vi "ClassPanel.vi"(8 "error in (no error)":errorcluster caption="entrée d'erreur (pas d'erreur)", 11 "SymphonyCCD.lvclass":refnum<class "SymphonyCCD.lvclass">) -> (0 "error out":errorcluster caption="sortie d'erreur", 3 "SymphonyCCD.lvclass Out":refnum<class "SymphonyCCD.lvclass">)   [LabVIEW 2019, in "SymphonyCCD.lvclass"]
uses:
  SymphonyCCD.lvclass
  <userlib>/JY Symphony/NoiseCorr.ctl
  C:/Programmes Labview/LabscanV1A/DevicesClass/BaseDevice/BaseDevice.lvclass
  SymphonyCCD.lvclass/SymphonyCCD.ctl
  BaseDevice/ClassQueueMess.ctl
  <vilib>/Utility/miscctls.llb/LVStringsAndValuesArrayTypeDef_U16.ctl
  BaseDevice/Accessor/GetClassEvent.vi
panel:
  in  "Acq":bool
  in  "Tabs":T1(tab)
  in  "NoiseWindow":bool caption="Noise Window"
  in  "Continuous Acq":bool
  in  "IntegTime":u32=60 caption="Integration\nTime (ms)" min=10 max=100000 step=1
  in  "AquireImage":bool caption="MiseAJour"
  out "AcqTime":dbl caption="Acq. Time (s)" format="%#.3f"
  in  "ADC":u16(ring) caption="Device Name" items=["ADC1:  20 kHz Tab 1", "ADC1:  50 kHz Tab 2"]
  in  "Gain":u16(ring) caption="Device Name" items=["Gain  0.6(x)"=10, "Gain  1.0(x)"=11, "Gain  2.0(x)"=12, "Gain  4.0(x)"=13, "Gain  6.7(x)"=8, "Gain 13.3(x)"=2]
  out "Temp °C":dbl
  in  "Shutter Enable":bool=TRUE
  out "Aquiring":bool
  in  "Save Data":bool caption="Save\nData"
  in  "Clear Graph":bool caption="Clear\nGraph"
  in  "Graph Number":i32 min=0 max=256 step=1
  in  "Image Mode":bool=TRUE
  in  "Accumulation":u16=1 min=1 max=256 step=1
  in  "Noise Mode":T2=enum."One For Every Acq"
  in  "Y End":i32=256 min=2 max=256 step=1
  out "areas":i32[][](array[numeric])=[[1], [1], [1], [1024], [256], [1], [256]]
  in  "Y Bins":i32=1 min=1 max=256 step=1
  in  "X Start":i32=1 min=1 max=1023 step=1
  in  "X End":i32=1024 min=2 max=1024 step=1
  in  "Y Start":i32=1 min=1 max=255 step=1
  in  "SetAreas":bool caption="MiseAJour"
  in  "Max Find Rng":bool
  in  "Window AvgSamp":u32=1 caption="Window Avg Samples" min=1 step=1
  in  "Window width":dbl=1.0 caption="Window Width(sigma)"
  in  "MultSource":u16(ring) caption="Multiplier Source"
  in  "MaxFindEnd":dbl caption="End (nm)"
  in  "LambdaOffset":dbl caption="Lambda(nm) Offset"
  in  "MaxFindStart":dbl caption="Start (nm)"
  in  "SetConv":bool caption="MiseAJour"
  in  "Wavelength Source":u16(ring)
  in  "MainProgQ":refnum<queue>
  in  "MainProgQEvent":refnum<user-event>
  in  "Stop":bool
  out "Init Program":bool
  # "Symphony Camera"
  # "this MUST labeled with class name"
  # "this MUST be present and labeled \"Stop\""
  # "Single Acq"
  # "Wavelenght Conversion Settings"
  # "Noise Filtering Settings"
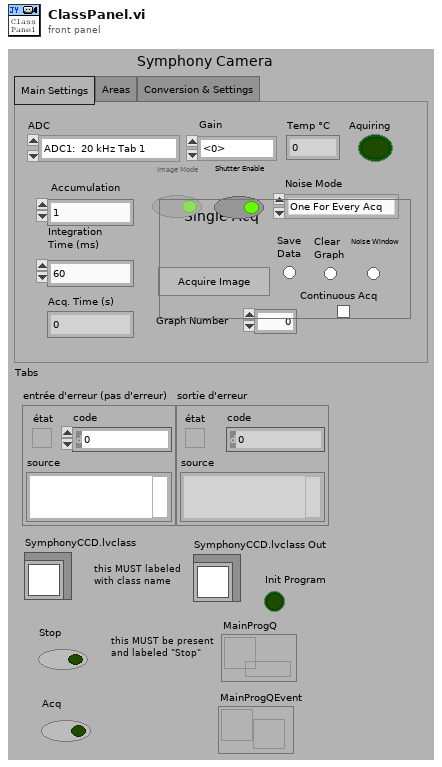
[diagram p1: front panel]
types:
  T1 = enum32{"Main Settings", "Areas", "Conversion & Settings"}
  T2 = typedef "NoiseCorr.ctl" = enum16{"Off", "One For All Acq", "One For Every Acq"}
  T3 = cluster{"Message":string, "Data":variant, "Code":i32}
  T4 = typedef "LVStringsAndValuesArrayTypeDef_U16.ctl" = cluster{"String":string, "Value":u16}[]
  T5 = cluster{"Chaînes et valeurs []":T4, u16, "Chaînes et valeurs [] 2":T4, u16, i16, i32[][], dbl, bool, bool, u16, u16}
  T6 = typedef "ClassQueueMess.ctl" = u16
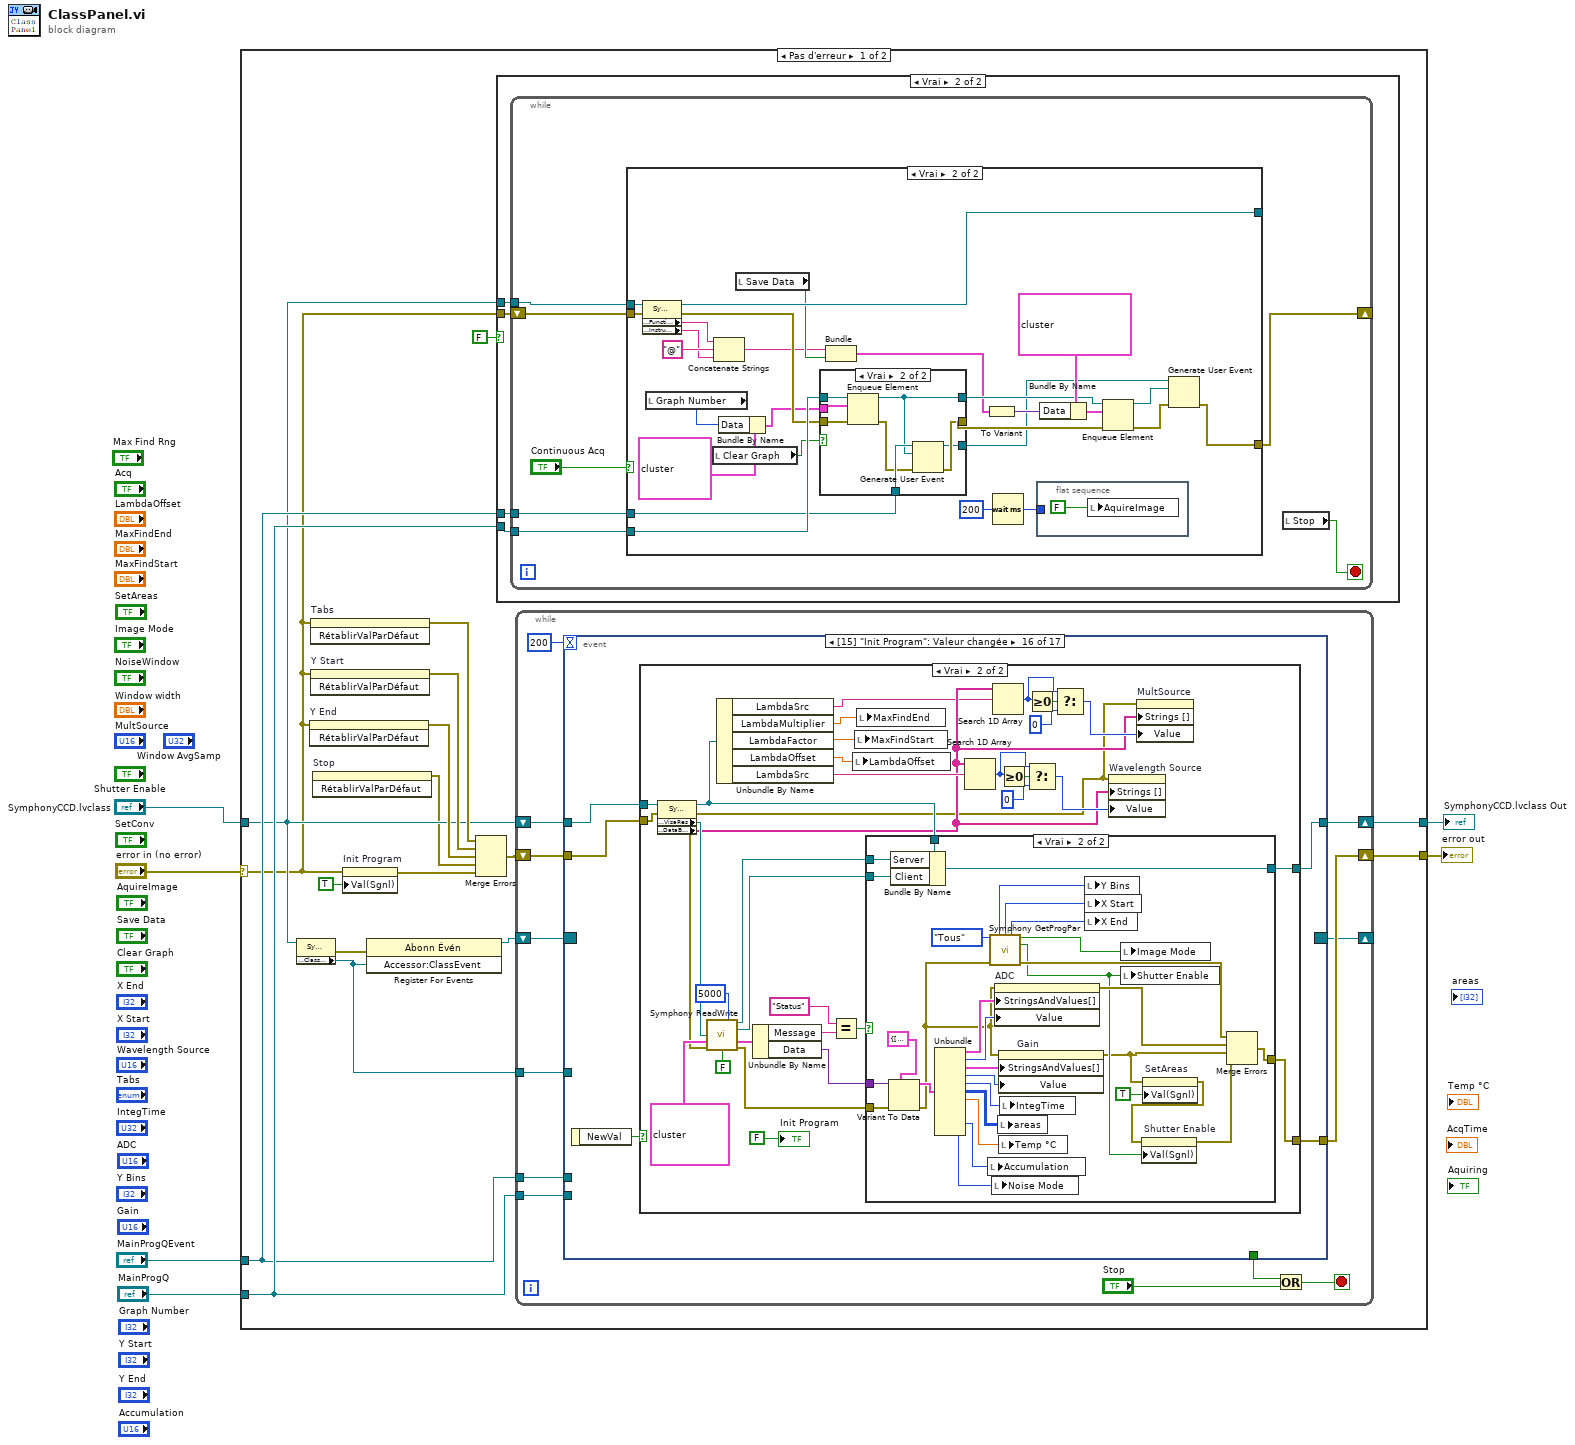
[diagram p0: block diagram]
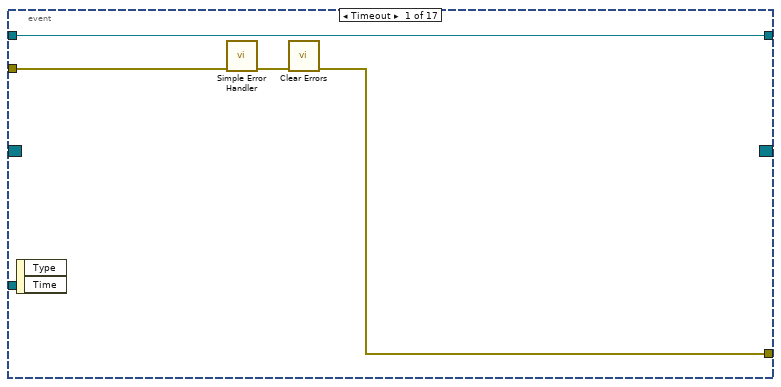
[diagram p5: hidden frame]
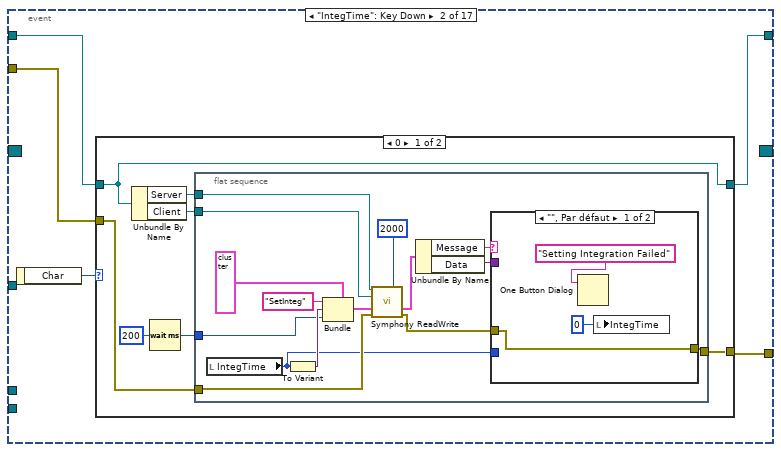
[diagram p6: hidden frame]
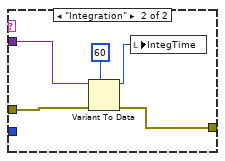
[diagram p7: hidden frame]
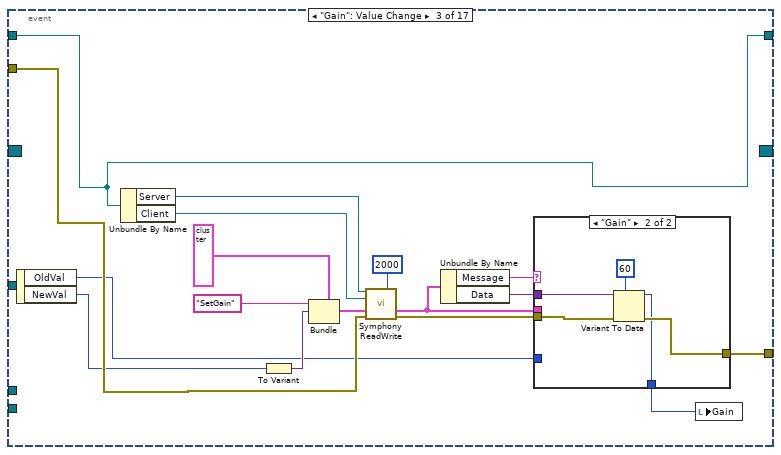
[diagram p9: hidden frame]
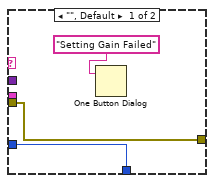
[diagram p10: hidden frame]
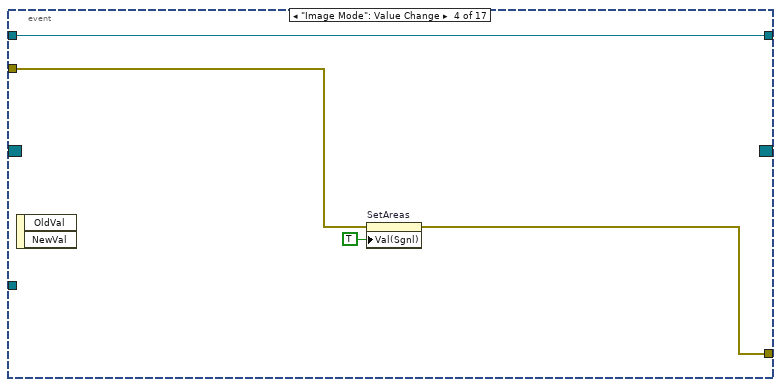
[diagram p11: hidden frame]
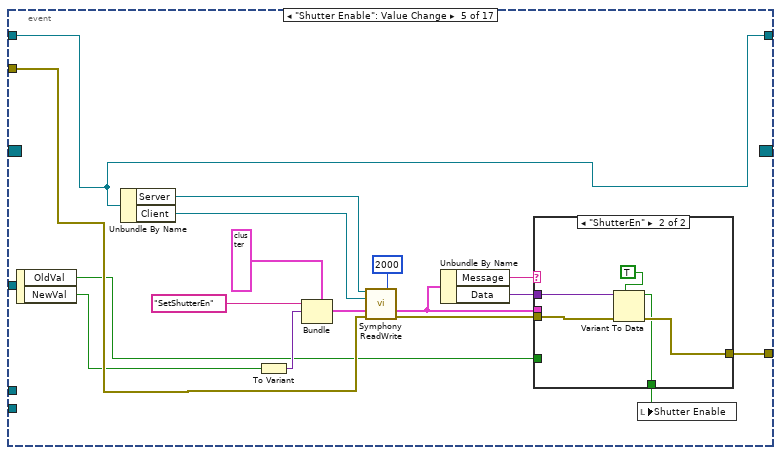
[diagram p12: hidden frame]
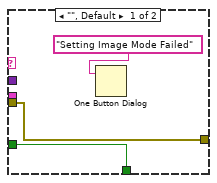
[diagram p13: hidden frame]
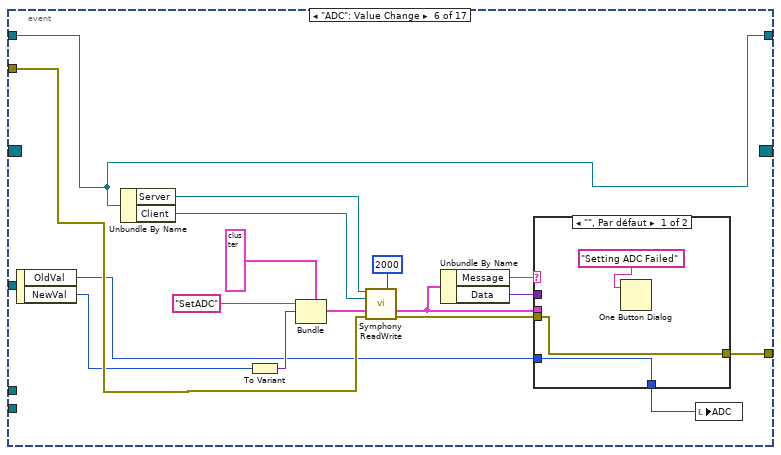
[diagram p14: hidden frame]
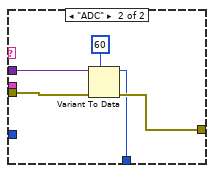
[diagram p15: hidden frame]
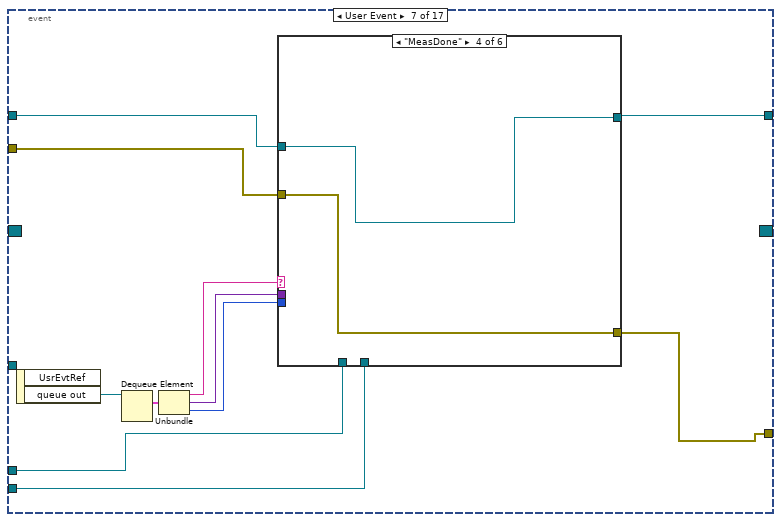
[diagram p16: hidden frame]
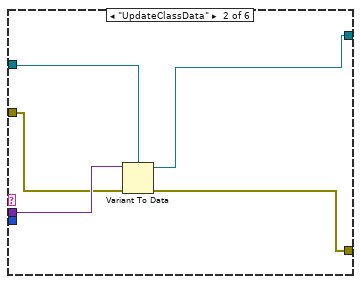
[diagram p18: hidden frame]
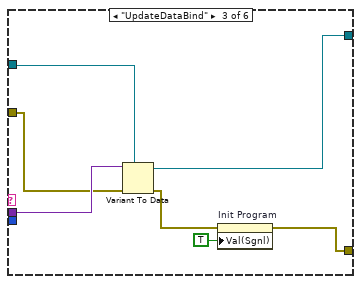
[diagram p19: hidden frame]
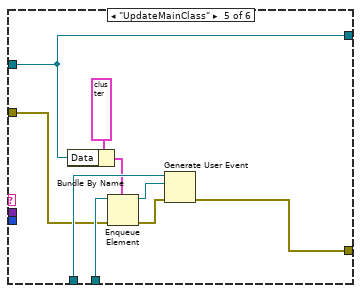
[diagram p20: hidden frame]
diagram:
  n1 = case shown="Pas d'erreur" "error in (no error)" {
    selector: "error in (no error)" -> [w9 w587]
    tunnel: [w23 w587] -> w5
    tunnel: "SymphonyCCD.lvclass" -> [w12 w586]
    tunnel: [w22 w586] -> w3
    tunnel: "MainProgQEvent" -> [w13 _]
    tunnel: "MainProgQ" -> [w14 _]
    frame No Error {
      n2 = property class="SymphonyCCD.lvclass"(reference=w12) -> (error out=w21:errorcluster, "Accessor:ClassEvent"=w19:refnum<user-event>)  [unwired: 1 in, 1 out]
      n3 = invoke on="Y End" class="NumNb (strict)" method="RétablirValParDéfaut"(error in=w9) -> (error out=w17:errorcluster)  [unwired: 2 in, 2 out]
      n4 = invoke on="Tabs" class="TabCtl (strict)" method="RétablirValParDéfaut"(error in=w9) -> (error out=w15:errorcluster)  [unwired: 2 in, 2 out]
      n5 = invoke on="Y Start" class="NumNb (strict)" method="RétablirValParDéfaut"(error in=w9) -> (error out=w16:errorcluster)  [unwired: 2 in, 2 out]
      n6 = invoke on="Stop" class="Bool (strict)" method="RétablirValParDéfaut"() -> (error out=w10:errorcluster)  [unwired: 3 in, 2 out]
      n7 = property on="Init Program" class="Bool (strict)"(error in=w9, "Val(Sgnl)"=TRUE ("Valeur (Signalisation)")) -> (error out=w8:errorcluster)  [unwired: 1 in, 1 out]
      n8 = register-events(error in=w21, w19) -> (reference out=w20:refnum<event-registration>)  [unwired: 1 in, 1 out]
      n9 = Merge Errors(w15, w16, w17, w10, w8) -> (w18:errorcluster)
      n10 = case shown="Vrai" FALSE {
        tunnel: w9 -> [_ w27]
        tunnel: w14 -> [_ w26]
        tunnel: w13 -> [_ w25]
        tunnel: w12 -> [_ w24]
        frame False {
        }
        frame True {
          n11 = while {
            shift-right: [w30] -> _
            shift-left: w27 -> [w33]
            tunnel: w25 -> [w32]
            tunnel: w26 -> [w31]
            tunnel: w24 -> [w29]
            stop <- w28 stop-if-true
            n12 = case shown="Vrai" "Continuous Acq" {
              tunnel: w29 -> [w36 w63]
              tunnel: w32 -> [_ w38]
              tunnel: w31 -> [_ w48]
              tunnel: [w36 w61] -> _
              tunnel: w33 -> [w35 w56]
              tunnel: [w35 w55] -> w30
              frame False {
              }
              frame True {
                n13 = property class="SymphonyCCD.lvclass"(reference=w63, error in=w56) -> (reference out=w61:refnum<class "SymphonyCCD.lvclass">, error out=w46:errorcluster, "Accessor:Function"=w54:string, "Accessor:InstrumentName"=w52:string)
                n14 = local read "Graph Number"() -> (w39:i32)
                n15 = local read "Clear Graph"() -> (w40:bool)
                n16 = Concatenate Strings(w54, "@" ("chaîne"), w52) -> (w41:string)
                n17 = Bundle By Name(cluster=cluster{"Message":string, "Data":variant, i32} {"Message"="ClearGraph", "Data"=variant, 0} ("élément"), "Data"=w39) -> (w42:cluster{"Message":string, "Data":variant, i32})
                n18 = local read "Save Data"() -> (w45:bool)
                n19 = case shown="Vrai" w40 {
                  tunnel: [w66 w69] -> w49
                  tunnel: w48 -> [w65 w74]
                  tunnel: [w65 w67] -> w47
                  tunnel: w46 -> [w66 w73]
                  tunnel: w42 -> [_ w72]
                  tunnel: w38 -> [w64 w71]
                  tunnel: [w64 w68] -> w37
                  frame False {
                  }
                  frame True {
                    n20 = Enqueue Element(queue=w74, element=w72, error in (no error)=w73) -> (queue out=w67:refnum<queue>, error out=w70:errorcluster)  [unwired: 1 in, 1 out]
                    n21 = Generate User Event(user event=w71, event data cluster=w67, error in=w70) -> (user event out=w68:refnum<user-event>, error out=w69:errorcluster)  [unwired: 1 in]
                  }
                }
                n22 = Bundle(w41, "Save Data"=w45) -> (w44:cluster{string, "Save Data":bool})  [unwired: 1 in]
                n23 = To Variant(anything=w44) -> (Variant=w59:variant)
                n24 = Wait (ms)(milliseconds to wait=u32 200 ("attente (ms)")) -> (millisecond timer value=w51:u32)
                n25 = flat-sequence {
                  tunnel: w51 -> [_]
                  frame #0 {
                    n26 = local write "AquireImage"(FALSE) -> ()
                  }
                }
                n27 = Bundle By Name(cluster=cluster{"Message":string, "Data":variant, i32} {"Message"="ArrayDevAcqSetup", "Data"=variant, 0} ("élément"), "Data"=w59) -> (w58:cluster{"Message":string, "Data":variant, i32})
                n28 = Enqueue Element(queue=w47, element=w58, error in (no error)=w49) -> (queue out=w62:refnum<queue>, error out=w57:errorcluster)  [unwired: 1 in, 1 out]
                n29 = Generate User Event(user event=w37, event data cluster=w62, error in=w57) -> (error out=w55:errorcluster)  [unwired: 1 in, 1 out]
              }
            }
            n30 = local read "Stop"() -> (w28:bool)
          }
        }
      }
      n31 = while {
        shift-right: [w86] -> w23
        shift-left: w18 -> [w87]
        shift-right: [w83] -> w22
        shift-left: w12 -> [w85]
        shift-right: [w80] -> _
        shift-left: w20 -> [w77]
        tunnel: w13 -> [w79]
        tunnel: w14 -> [w78]
        tunnel: w19 -> [w76]
        stop <- w82 stop-if-true
        n32 = event shown="[15] \"Init Program\": Valeur changée" {
          selector: w77 -> [_ _ _ _ _ _ _ _ _ _ _ _ _ _ _ _ _]
          dyn-events: [_ _ _ _ _ _ _ _ _ _ _ _ _ _ _ _ _] -> w80
          timeout: 200 -> [_ _ _ _ _ _ _ _ _ _ _ _ _ _ _ _ _]
          tunnel: w87 -> [w91 w95 w146 w157 w175 w200 w218 w253 w262 w321 w365 w394 w409 w413 w461 w488 w561]
          tunnel: [w89 w93 w144 w156 w173 w198 w212 w251 w261 w320 w388 w407 w409 w412 w460 w487 w559] -> w86
          tunnel: w85 -> [w92 w96 w145 w158 w174 w199 w219 w257 w260 w319 w364 w397 w408 w417 w463 w486 w562]
          tunnel: [_ _ _ _ _ _ _ _ _ _ _ _ TRUE _ _ _ _] -> w84
          tunnel: [w92 w94 w145 w158 w174 w199 w211 w254 w259 w318 w387 w406 w408 w414 w462 w485 w560] -> w83
          tunnel: w79 -> [_ _ _ _ _ _ w210 _ _ _ _ _ _ w416 _ _ _]
          tunnel: w78 -> [_ _ _ _ _ _ w209 _ _ _ _ _ _ w415 _ _ _]
          tunnel: w76 -> [_ _ _ _ _ _ _ _ w263 w322 _ _ _ _ _ _ _]
          event Timeout {
            n33 = event-data() -> ()  [unwired: 1 in, 2 out]
            n34 = call <vilib>:"Simple Error Handler.vi"("error in (no error)"=w91) -> ("error out"=w90:errorcluster)  [unwired: 4 in, 4 out]
            n35 = call <vilib>:"Clear Errors.vi"("error in (no error)"=w90) -> ("error out"=w89:errorcluster)  [unwired: 5 in, 1 out]
          }
          event "IntegTime": Key Down {
            n36 = event-data() -> ("Char"=w97:i16)  [unwired: 1 in]
            n37 = case shown="0" w97 {
              tunnel: w96 -> [w101 w129]
              tunnel: w95 -> [w100 w128]
              tunnel: [w101 w129] -> w94
              tunnel: [w104 w128] -> w93
              frame 0 {
                n38 = Unbundle By Name(w101) -> ("Server"=w103:refnum<k13>, "Client"=w102:refnum<k13>)
                n39 = Wait (ms)(milliseconds to wait=u32 200 ("attente (ms)")) -> (millisecond timer value=w99:u32)
                n40 = flat-sequence {
                  tunnel: [w109] -> w104
                  tunnel: w103 -> [w114]
                  tunnel: w102 -> [w113]
                  tunnel: w100 -> [w112]
                  tunnel: w99 -> [w111]
                  frame #0 {
                    n41 = local read "IntegTime"() -> (w107:u32)
                    n42 = To Variant(anything=w107) -> (Variant=w115:variant)
                    n43 = Bundle(cluster=T3 {"Message"="", "Data"=variant, "Code"=0} ("Message In"), "Message"="SetInteg", "Data"=w115, "Code"=w111) -> (w117:T3)
                    n44 = call <userlib>:"Symphony ReadWrite.vi"("ServerIn"=w114, "Read timeout ms(10000)"=2000, "ClientIn"=w113, "Message In"=w117, "ErrorIn (no error)"=w112) -> ("Data Out"=w110:T3, "error out"=w108:errorcluster)  [unwired: 7 in, 2 out]
                    n45 = Unbundle By Name(w110) -> ("Message"=w106:string, "Data"=w105:variant)
                    n46 = case shown="\"\", Par défaut" w106 {
                      tunnel: [w122 w127] -> w109
                      tunnel: w108 -> [w122 w126]
                      tunnel: w107 -> [_ _]
                      tunnel: w105 -> [_ w124]
                      frame "", Default {
                        n47 = One Button Dialog(message="Setting Integration Failed") -> ()  [unwired: 1 in, 1 out]
                        n48 = local write "IntegTime"(u32 0 ("IntegTime")) -> ()
                      }
                      frame "Integration" {
                        n49 = Variant To Data(error in=w126, type=u32 60 ("IntegTime"), Variant=w124) -> (data=w123:u32, error out=w127:errorcluster)
                        n50 = local write "IntegTime"(w123) -> ()
                      }
                    }
                  }
                }
              }
              frame Default {
              }
            }
          }
          event "Gain": Value Change {
            n51 = event-data() -> ("OldVal"=w133:u16, "NewVal"=w141:u16)  [unwired: 1 in]
            n52 = Unbundle By Name(w145) -> ("Server"=w143:refnum<k13>, "Client"=w142:refnum<k13>)
            n53 = To Variant(anything=w141) -> (Variant=w136:variant)
            n54 = Bundle(cluster=T3 {"Message"="", "Data"=variant, "Code"=0} ("Message In"), "Message"="SetGain", "Data"=w136) -> (w138:T3)  [unwired: 1 in]
            n55 = call <userlib>:"Symphony ReadWrite.vi"("ServerIn"=w143, "Read timeout ms(10000)"=2000, "ClientIn"=w142, "Message In"=w138, "ErrorIn (no error)"=w146) -> ("Data Out"=w132:T3, "error out"=w135:errorcluster)  [unwired: 7 in, 2 out]
            n56 = Unbundle By Name(w132) -> ("Message"=w131:string, "Data"=w130:variant)
            n57 = case shown="\"Gain\"" w131 {
              tunnel: [w148 w154] -> w144
              tunnel: w132 -> [_ _]
              tunnel: w135 -> [w148 w153]
              tunnel: [w149 w151] -> w134
              tunnel: w133 -> [w149 _]
              tunnel: w130 -> [_ w150]
              frame "", Default {
                n58 = One Button Dialog(message="Setting Gain Failed") -> ()  [unwired: 1 in, 1 out]
              }
              frame "Gain" {
                n59 = Variant To Data(error in=w153, type=u16 60 ("IntegTime"), Variant=w150) -> (data=w151:u16, error out=w154:errorcluster)
              }
            }
            n60 = local write "Gain"(w134) -> ()
          }
          event "Image Mode": Value Change {
            n61 = event-data() -> ()  [unwired: 1 in, 2 out]
            n62 = property on="SetAreas" class="Bool (strict)"(error in=w157, "Val(Sgnl)"=TRUE ("Valeur (Signalisation)")) -> (error out=w156:errorcluster)  [unwired: 1 in, 1 out]
          }
          event "Shutter Enable": Value Change {
            n63 = event-data() -> ("OldVal"=w162:bool, "NewVal"=w170:bool)  [unwired: 1 in]
            n64 = Unbundle By Name(w174) -> ("Server"=w172:refnum<k13>, "Client"=w171:refnum<k13>)
            n65 = To Variant(anything=w170) -> (Variant=w165:variant)
            n66 = Bundle(cluster=T3 {"Message"="", "Data"=variant, "Code"=0} ("Message In"), "Message"="SetShutterEn", "Data"=w165) -> (w167:T3)  [unwired: 1 in]
            n67 = call <userlib>:"Symphony ReadWrite.vi"("ServerIn"=w172, "Read timeout ms(10000)"=2000, "ClientIn"=w171, "Message In"=w167, "ErrorIn (no error)"=w175) -> ("Data Out"=w161:T3, "error out"=w164:errorcluster)  [unwired: 7 in, 2 out]
            n68 = Unbundle By Name(w161) -> ("Message"=w160:string, "Data"=w159:variant)
            n69 = case shown="\"ShutterEn\"" w160 {
              tunnel: [w177 w183] -> w173
              tunnel: w161 -> [_ _]
              tunnel: w164 -> [w177 w182]
              tunnel: [w178 w181] -> w163
              tunnel: w162 -> [w178 _]
              tunnel: w159 -> [_ w180]
              frame "", Default {
                n70 = One Button Dialog(message="Setting Image Mode Failed") -> ()  [unwired: 1 in, 1 out]
              }
              frame "ShutterEn" {
                n71 = Variant To Data(error in=w182, type=TRUE, Variant=w180) -> (data=w181:bool, error out=w183:errorcluster)
              }
            }
            n72 = local write "Shutter Enable"(w163) -> ()
          }
          event "ADC": Value Change {
            n73 = event-data() -> ("OldVal"=w187:u16, "NewVal"=w195:u16)  [unwired: 1 in]
            n74 = Unbundle By Name(w199) -> ("Server"=w197:refnum<k13>, "Client"=w196:refnum<k13>)
            n75 = To Variant(anything=w195) -> (Variant=w190:variant)
            n76 = Bundle(cluster=T3 {"Message"="", "Data"=variant, "Code"=0} ("Message In"), "Message"="SetADC", "Data"=w190) -> (w192:T3)  [unwired: 1 in]
            n77 = call <userlib>:"Symphony ReadWrite.vi"("ServerIn"=w197, "Read timeout ms(10000)"=2000, "ClientIn"=w196, "Message In"=w192, "ErrorIn (no error)"=w200) -> ("Data Out"=w186:T3, "error out"=w189:errorcluster)  [unwired: 7 in, 2 out]
            n78 = Unbundle By Name(w186) -> ("Message"=w185:string, "Data"=w184:variant)
            n79 = case shown="\"\", Par défaut" w185 {
              tunnel: [w202 w208] -> w198
              tunnel: w186 -> [_ _]
              tunnel: w189 -> [w202 w207]
              tunnel: [w203 w205] -> w188
              tunnel: w187 -> [w203 _]
              tunnel: w184 -> [_ w204]
              frame "", Default {
                n80 = One Button Dialog(message="Setting ADC Failed") -> ()  [unwired: 1 in, 1 out]
              }
              frame "ADC" {
                n81 = Variant To Data(error in=w207, type=u16 60 ("IntegTime"), Variant=w204) -> (data=w205:u16, error out=w208:errorcluster)
              }
            }
            n82 = local write "ADC"(w188) -> ()
          }
          event User Event {
            n83 = event-data() -> ("queue out"=w216:refnum<queue>)  [unwired: 1 in, 1 out]
            n84 = Dequeue Element(queue=w216) -> (element=w217:cluster{"Message":string, "Data":variant, i32})  [unwired: 2 in, 3 out]
            n85 = Unbundle(w217) -> ("Message"=w215:string, "Data"=w214:variant, w213:i32)
            n86 = case shown="\"MeasDone\"" w215 {
              tunnel: w218 -> [w221 w224 w231 w235 w238 w248]
              tunnel: w214 -> [_ w226 w233 _ _ _]
              tunnel: w219 -> [w220 w225 w232 w234 w236 w247]
              tunnel: [w220 w222 w230 w234 w236 w247] -> w211
              tunnel: [w221 w223 w228 w235 w237 w246] -> w212
              tunnel: w213 -> [_ _ _ _ _ _]
              tunnel: w210 -> [_ _ _ _ w242 _]
              tunnel: w209 -> [_ _ _ _ w241 _]
              frame Default {
              }
              frame "UpdateClassData" {
                n87 = Variant To Data(error in=w224, type=w225, Variant=w226) -> (data=w222:refnum<class "SymphonyCCD.lvclass">, error out=w223:errorcluster)
              }
              frame "UpdateDataBind" {
                n88 = Variant To Data(error in=w231, type=w232, Variant=w233) -> (data=w230:refnum<class "SymphonyCCD.lvclass">, error out=w229:errorcluster)
                n89 = property on="Init Program" class="Bool (strict)"(error in=w229, "Val(Sgnl)"=TRUE ("Valeur (Signalisation)")) -> (error out=w228:errorcluster)  [unwired: 1 in, 1 out]
              }
              frame "MeasDone" {
              }
              frame "UpdateMainClass" {
                n90 = Bundle By Name(cluster=cluster{"Message":string, "Data":variant, i32} {"Message"="", "Data"=variant, 0} ("élément"), "Data"=w236) -> (w239:cluster{"Message":string, "Data":variant, i32})
                n91 = Enqueue Element(queue=w241, element=w239, error in (no error)=w238) -> (queue out=w244:refnum<queue>, error out=w243:errorcluster)  [unwired: 1 in, 1 out]
                n92 = Generate User Event(user event=w242, event data cluster=w244, error in=w243) -> (error out=w237:errorcluster)  [unwired: 1 in, 1 out]
              }
              frame "ShowDiag" {
                n93 = control-ref of="Ce VI"() -> (w245:refnum<vi>)
                n94 = call <userlib>:"AnimExecGen.vi"("ErrorIn(No Error)"=w248, "Animer l'exécution ?"=TRUE, "ViRef"=w245) -> ("sortie d'erreur"=w246:errorcluster)  [unwired: 8 in]
              }
            }
          }
          event "Save Data": Value Change {
            w250 = T6 1 items=["UpdateClassData", "UpdateMainClass", "UpdateDataBind"] ("Menu déroulant")
            n95 = event-data() -> ("NewVal"=w256:bool)  [unwired: 1 in, 5 out]
            n96 = property class="SymphonyCCD.lvclass"(reference=w257, error in=w253, "Accessor:SaveArrDat"=w256) -> (reference out=w255:refnum<class "SymphonyCCD.lvclass">, error out=w252:errorcluster)
            n97 = call-dynamic "SetClassQueueMessage.vi"("ErrorIn(No Error)"=w252, "Menu déroulant"=w250, "Symphony.lvclass"=w255) -> ("sortie d'erreur"=w251:errorcluster, "Symphony.lvclass Out"=w254:refnum<class "SymphonyCCD.lvclass">)  [unwired: 7 in]
          }
          event "SetAreas": Value Change {
            n98 = event-data() -> ("NewVal"=w258:bool)  [unwired: 1 in]
            n99 = case shown="Vrai" w258 {
              tunnel: [w305 w316] -> w259
              tunnel: w263 -> [_ _]
              tunnel: w262 -> [w270 w315]
              tunnel: [w288 w315] -> w261
              tunnel: w260 -> [w269 w316]
              frame True {
                w267 = T6 1 items=["UpdateClassData", "UpdateMainClass"] ("Menu déroulant")
                n100 = local read "Accumulation"() -> (w273:u16)
                n101 = local read "Noise Mode"() -> (w271:T2)
                n102 = local read "NoiseWindow"() -> (w272:bool)
                n103 = local read "Y Start"() -> (w301:i32)
                n104 = local read "Image Mode"() -> (w274:bool)
                n105 = local read "Y Bins"() -> (w278:i32)
                n106 = local read "X End"() -> (w291:i32)
                n107 = local read "X Start"() -> (w302:i32)
                n108 = local read "Y End"() -> (w292:i32)
                n109 = Tick Count (ms)() -> (millisecond timer value=w281:u32)
                n110 = Unbundle By Name(w269) -> ("Server"=w293:refnum<k13>, "Client"=w294:refnum<k13>)
                n111 = call-dynamic "SetClassQueueMessage.vi"("ErrorIn(No Error)"=w270, "Menu déroulant"=w267, "Symphony.lvclass"=w269) -> ("sortie d'erreur"=w266:errorcluster, "Symphony.lvclass Out"=w268:refnum<class "SymphonyCCD.lvclass">)  [unwired: 7 in]
                n112 = call <userlib>:"Symphony Format AreaV2.vi"("Y Start"=w301, "Y End"=w292, "ImageMode"=w274, "error in (no error)"=w266, "X Start"=w302, "X End"=w291, "numAreas"=w278) -> ("error out"=w290:errorcluster, "areas :"=w280:i32[][], "X Size Out"=w300:i32)  [unwired: 1 in]
                n113 = Bundle("areas :"=w280, "Image Mode"=w274) -> (w279:cluster{"areas :":i32[][], "Image Mode":bool})  [unwired: 1 in]
                n114 = To Variant(anything=w279) -> (Variant=w298:variant)
                n115 = for {
                  N: w300 -> [_]
                  tunnel: w302 -> [w314]
                  tunnel: [w312] -> w304 mode=indexing
                  i -> [w311]
                  n116 = Add(x=w314, y=w311) -> (x+y=w313:i32)
                  n117 = To Double Precision Float(number=w313) -> (double precision float=w312:dbl)
                }
                n118 = Bundle By Name(cluster=w268, "Y Size"=w278) -> (w303:refnum<class "SymphonyCCD.lvclass">)
                n119 = Bundle(cluster=T3 {"Message"="", "Data"=variant, "Code"=0} ("Message In"), "Message"="SetArea", "Data"=w298, "Code"=w281) -> (w299:T3)
                n120 = call <userlib>:"Symphony Format CrvNames.vi"("Noise Mode"=w271, "NoiseWindow"=w272, "error in (no error)"=w266, "Accumulation"=w273, "numAreas"=w278) -> ("error out"=w277:errorcluster, "DatDisplayNm"=w264:string[], "VarParY"=w275:dbl[], "SubDatDisplayNm"=w276:string[])  [unwired: 2 in]
                n121 = call <userlib>:"Symphony ReadWrite.vi"("ServerIn"=w293, "Read timeout ms(10000)"=2000, "ClientIn"=w294, "Message In"=w299, "ErrorIn (no error)"=w290) -> ("Data Out"=w289:T3, "error out"=w284:errorcluster)  [unwired: 7 in, 2 out]
                n122 = Unbundle By Name(w289) -> ("Message"=w287:string, "Data"=w286:variant)
                n123 = property class="SymphonyCCD.lvclass"(reference=w303, error in=w266, "Accessor:SubDatDisplayNm"=w276, "Accessor:SubScanTable(y)"=w275, "Accessor:ScanTable"=w304, "Accessor:ArrayDatNm"=w264) -> (reference out=w305:refnum<class "SymphonyCCD.lvclass">, error out=w265:errorcluster)
                n124 = Wait (ms)(milliseconds to wait=u32 200 ("attente (ms)")) -> (millisecond timer value=w282:u32)
                n125 = case shown="Par défaut" w287 {
                  tunnel: w286 -> [_ _]
                  tunnel: [w307 w310] -> w285
                  tunnel: w284 -> [w307 w310]
                  tunnel: w280 -> [_ w309]
                  frame Default {
                    n126 = One Button Dialog(message="Error Setting Areas" ("Message")) -> ()  [unwired: 1 in, 1 out]
                  }
                  frame "Area" {
                    n127 = local write "areas"(w309) -> ()
                  }
                }
                n128 = flat-sequence {
                  tunnel: w282 -> [_]
                  frame #0 {
                    n129 = local write "SetAreas"(FALSE) -> ()
                  }
                }
                n130 = Merge Errors(w265, w277, w285) -> (w288:errorcluster)
              }
              frame False {
              }
            }
          }
          event "Accumulation": Key Down {
            n131 = event-data() -> ("Char"=w317:i16)  [unwired: 1 in]
            n132 = case shown="0" w317 {
              tunnel: [w353 w359] -> w318
              tunnel: w322 -> [_ _]
              tunnel: w321 -> [w328 w358]
              tunnel: [w344 w358] -> w320
              tunnel: w319 -> [w327 w359]
              frame 0 {
                w329 = T6 1 items=["UpdateClassData", "UpdateMainClass"] ("Menu déroulant")
                n133 = Wait (ms)(milliseconds to wait=u32 200 ("attente (ms)")) -> (millisecond timer value=w333:u32)
                n134 = local read "NoiseWindow"() -> (w335:bool)
                n135 = local read "Y Bins"() -> (w334:i32)
                n136 = flat-sequence {
                  tunnel: [w354] -> w330
                  tunnel: w333 -> [_]
                  frame #0 {
                    n137 = local read "Accumulation"() -> (w354:u16)
                  }
                }
                n138 = Unbundle By Name(w327) -> ("Server"=w346:refnum<k13>, "Client"=w347:refnum<k13>)
                n139 = Tick Count (ms)() -> (millisecond timer value=w339:u32)
                n140 = call-dynamic "SetClassQueueMessage.vi"("ErrorIn(No Error)"=w328, "Menu déroulant"=w329, "Symphony.lvclass"=w327) -> ("sortie d'erreur"=w324:errorcluster, "Symphony.lvclass Out"=w326:refnum<class "SymphonyCCD.lvclass">)  [unwired: 7 in]
                n141 = To Variant(anything=w330) -> (Variant=w351:variant)
                n142 = Bundle(cluster=T3 {"Message"="", "Data"=variant, "Code"=0} ("Message In"), "Message"="SetAcc", "Data"=w351, "Code"=w339) -> (w352:T3)
                n143 = call <userlib>:"Symphony Format CrvNames.vi"("Noise Mode"="Noise Mode", "NoiseWindow"=w335, "error in (no error)"=w324, "Accumulation"=w330, "numAreas"=w334) -> ("error out"=w338:errorcluster, "DatDisplayNm"=w323:string[], "VarParY"=w336:dbl[], "SubDatDisplayNm"=w337:string[])  [unwired: 2 in]
                n144 = call <userlib>:"Symphony ReadWrite.vi"("ServerIn"=w346, "Read timeout ms(10000)"=2000, "ClientIn"=w347, "Message In"=w352, "ErrorIn (no error)"=w324) -> ("Data Out"=w345:T3, "error out"=w340:errorcluster)  [unwired: 7 in, 2 out]
                n145 = Unbundle By Name(w345) -> ("Message"=w343:string, "Data"=w342:variant)
                n146 = property class="SymphonyCCD.lvclass"(reference=w326, error in=w324, "Accessor:SubDatDisplayNm"=w337, "Accessor:SubScanTable(y)"=w336, "Accessor:ArrayDatNm"=w323) -> (reference out=w353:refnum<class "SymphonyCCD.lvclass">, error out=w325:errorcluster)
                n147 = case shown="Par défaut" w343 {
                  tunnel: w342 -> [_ _]
                  tunnel: [w355 w357] -> w341
                  tunnel: w340 -> [w355 w357]
                  frame Default {
                    n148 = One Button Dialog(message="Error Setting Accumulation" ("Message")) -> ()  [unwired: 1 in, 1 out]
                  }
                  frame "Accumulation" {
                  }
                }
                n149 = Merge Errors(w325, w338, w341) -> (w344:errorcluster)
              }
              frame Default {
              }
            }
          }
          event Value Change {
            w366 = T6 1 items=["UpdateClassData", "UpdateMainClass"] ("Menu déroulant")
            n150 = event-data() -> ("NewVal"=w367:T2)  [unwired: 1 in]
            n151 = local read "NoiseWindow"() -> (w370:bool)
            n152 = local read "Y Bins"() -> (w368:i32)
            n153 = local read "Accumulation"() -> (w369:u16)
            n154 = Unbundle By Name(w364) -> ("Server"=w380:refnum<k13>, "Client"=w381:refnum<k13>)
            n155 = Tick Count (ms)() -> (millisecond timer value=w374:u32)
            n156 = call-dynamic "SetClassQueueMessage.vi"("ErrorIn(No Error)"=w365, "Menu déroulant"=w366, "Symphony.lvclass"=w364) -> ("sortie d'erreur"=w362:errorcluster, "Symphony.lvclass Out"=w363:refnum<class "SymphonyCCD.lvclass">)  [unwired: 7 in]
            n157 = To Variant(anything=w367) -> (Variant=w385:variant)
            n158 = Bundle(cluster=T3 {"Message"="", "Data"=variant, "Code"=0} ("Message In"), "Message"="SetNoiseMode", "Data"=w385, "Code"=w374) -> (w386:T3)
            n159 = call <userlib>:"Symphony Format CrvNames.vi"("Noise Mode"=w367, "NoiseWindow"=w370, "error in (no error)"=w362, "Accumulation"=w369, "numAreas"=w368) -> ("error out"=w373:errorcluster, "DatDisplayNm"=w360:string[], "VarParY"=w371:dbl[], "SubDatDisplayNm"=w372:string[])  [unwired: 2 in]
            n160 = call <userlib>:"Symphony ReadWrite.vi"("ServerIn"=w380, "Read timeout ms(10000)"=2000, "ClientIn"=w381, "Message In"=w386, "ErrorIn (no error)"=w362) -> ("Data Out"=w379:T3, "error out"=w375:errorcluster)  [unwired: 7 in, 2 out]
            n161 = Unbundle By Name(w379) -> ("Message"=w378:string, "Data"=w377:variant)
            n162 = property class="SymphonyCCD.lvclass"(reference=w363, error in=w362, "Accessor:SubDatDisplayNm"=w372, "Accessor:SubScanTable(y)"=w371, "Accessor:ArrayDatNm"=w360) -> (reference out=w387:refnum<class "SymphonyCCD.lvclass">, error out=w361:errorcluster)
            n163 = case shown="\"NoiseMode\"" w378 {
              tunnel: w377 -> [_ _]
              tunnel: [w389 w391] -> w376
              tunnel: w375 -> [w389 w391]
              frame Default {
                n164 = One Button Dialog(message="Error Setting Accumulation" ("Message")) -> ()  [unwired: 1 in, 1 out]
              }
              frame "NoiseMode" {
              }
            }
            n165 = Merge Errors(w361, w373, w376) -> (w388:errorcluster)
          }
          event "NoiseWindow": Value Change {
            w398 = T6 1 items=["UpdateClassData", "UpdateMainClass"] ("Menu déroulant")
            n166 = event-data() -> ()  [unwired: 1 in, 1 out]
            n167 = local read "NoiseWindow"() -> (w402:bool)
            n168 = local read "Y Bins"() -> (w400:i32)
            n169 = local read "Accumulation"() -> (w401:u16)
            n170 = local read "Noise Mode"() -> (w399:T2)
            n171 = call-dynamic "SetClassQueueMessage.vi"("ErrorIn(No Error)"=w394, "Menu déroulant"=w398, "Symphony.lvclass"=w397) -> ("sortie d'erreur"=w395:errorcluster, "Symphony.lvclass Out"=w396:refnum<class "SymphonyCCD.lvclass">)  [unwired: 7 in]
            n172 = call <userlib>:"Symphony Format CrvNames.vi"("Noise Mode"=w399, "NoiseWindow"=w402, "error in (no error)"=w395, "Accumulation"=w401, "numAreas"=w400) -> ("error out"=w405:errorcluster, "DatDisplayNm"=w392:string[], "VarParY"=w403:dbl[], "SubDatDisplayNm"=w404:string[])  [unwired: 2 in]
            n173 = property class="SymphonyCCD.lvclass"(reference=w396, "Accessor:SubDatDisplayNm"=w404, "Accessor:SubScanTable(y)"=w403, "Accessor:ArrayDatNm"=w392) -> (reference out=w406:refnum<class "SymphonyCCD.lvclass">, error out=w393:errorcluster)  [unwired: 1 in]
            n174 = Merge Errors(w393, w405) -> (w407:errorcluster)
          }
          event Panel Close? {
            n175 = event-data() -> ()  [unwired: 1 in, 1 out]
            n176 = event-data("Discard?"=FALSE ("Rejeter ?")) -> ()  [unwired: 1 in, 1 out]
          }
          event "AquireImage": Value Change {
            n177 = event-data() -> ("NewVal"=w418:bool)  [unwired: 1 in]
            n178 = case shown="Vrai" w418 {
              tunnel: w417 -> [w420 w447]
              tunnel: w416 -> [_ w422]
              tunnel: w415 -> [_ w432]
              tunnel: [w420 w445] -> w414
              tunnel: w413 -> [w419 w440]
              tunnel: [w419 w439] -> w412
              frame False {
              }
              frame True {
                n179 = property class="SymphonyCCD.lvclass"(reference=w447, error in=w440) -> (reference out=w445:refnum<class "SymphonyCCD.lvclass">, error out=w430:errorcluster, "Accessor:Function"=w438:string, "Accessor:InstrumentName"=w436:string)
                n180 = local read "Graph Number"() -> (w423:i32)
                n181 = local read "Clear Graph"() -> (w424:bool)
                n182 = Concatenate Strings(w438, "@" ("chaîne"), w436) -> (w425:string)
                n183 = Bundle By Name(cluster=cluster{"Message":string, "Data":variant, i32} {"Message"="ClearGraph", "Data"=variant, 0} ("élément"), "Data"=w423) -> (w426:cluster{"Message":string, "Data":variant, i32})
                n184 = local read "Save Data"() -> (w429:bool)
                n185 = case shown="Vrai" w424 {
                  tunnel: [w450 w453] -> w433
                  tunnel: w432 -> [w449 w458]
                  tunnel: [w449 w451] -> w431
                  tunnel: w430 -> [w450 w457]
                  tunnel: w426 -> [_ w456]
                  tunnel: w422 -> [w448 w455]
                  tunnel: [w448 w452] -> w421
                  frame False {
                  }
                  frame True {
                    n186 = Enqueue Element(queue=w458, element=w456, error in (no error)=w457) -> (queue out=w451:refnum<queue>, error out=w454:errorcluster)  [unwired: 1 in, 1 out]
                    n187 = Generate User Event(user event=w455, event data cluster=w451, error in=w454) -> (user event out=w452:refnum<user-event>, error out=w453:errorcluster)  [unwired: 1 in]
                  }
                }
                n188 = Bundle(w425, "Save Data"=w429) -> (w428:cluster{string, "Save Data":bool})  [unwired: 1 in]
                n189 = To Variant(anything=w428) -> (Variant=w443:variant)
                n190 = Wait (ms)(milliseconds to wait=u32 200 ("attente (ms)")) -> (millisecond timer value=w435:u32)
                n191 = flat-sequence {
                  tunnel: w435 -> [_]
                  frame #0 {
                    n192 = local write "AquireImage"(FALSE) -> ()
                  }
                }
                n193 = Bundle By Name(cluster=cluster{"Message":string, "Data":variant, i32} {"Message"="ArrayDevAcqSetup", "Data"=variant, 0} ("élément"), "Data"=w443) -> (w442:cluster{"Message":string, "Data":variant, i32})
                n194 = Enqueue Element(queue=w431, element=w442, error in (no error)=w433) -> (queue out=w446:refnum<queue>, error out=w441:errorcluster)  [unwired: 1 in, 1 out]
                n195 = Generate User Event(user event=w421, event data cluster=w446, error in=w441) -> (error out=w439:errorcluster)  [unwired: 1 in, 1 out]
              }
            }
          }
          event "SetConv": Value Change {
            n196 = event-data() -> ("NewVal"=w464:bool)  [unwired: 1 in, 5 out]
            n197 = case shown="Vrai" w464 {
              tunnel: w463 -> [w466 w477]
              tunnel: [w466 w467] -> w462
              tunnel: w461 -> [w465 w469]
              tunnel: [w465 w468] -> w460
              frame False {
              }
              frame True {
                w471 = T6 1 items=["UpdateClassData", "UpdateMainClass"] ("Menu déroulant")
                n198 = property on="Wavelength Source" class="MDér (strict)"() -> ("Strings []"=w482:string[], "Value"=w483:u16)  [unwired: 2 in, 2 out]
                n199 = property on="MultSource" class="MDér (strict)"() -> ("Strings []"=w474:string[], "Value"=w473:u16)  [unwired: 2 in, 2 out]
                n200 = local read "MaxFindStart"() -> (w481:dbl)
                n201 = local read "LambdaOffset"() -> (w480:dbl)
                n202 = local read "MaxFindEnd"() -> (w476:dbl)
                n203 = Index Array(array=w482, index=w483) -> (element=w475:string)
                n204 = Index Array(array=w474, index=w473) -> (element=w472:string)
                n205 = Wait (ms)(milliseconds to wait=u32 500 ("attente (ms)")) -> (millisecond timer value=w479:u32)
                n206 = flat-sequence {
                  tunnel: w479 -> [_]
                  frame #0 {
                    n207 = local write "SetConv"(FALSE ("SetConv")) -> ()
                  }
                }
                n208 = Bundle By Name(cluster=w477, "LambdaMultiplier"=w476, "LambdaFactor"=w481, "LambdaOffset"=w480, "LambdaSrc"=w475, "MultiplierSrc"=w472) -> (w470:refnum<class "SymphonyCCD.lvclass">)
                n209 = call-dynamic "SetClassQueueMessage.vi"("ErrorIn(No Error)"=w469, "Menu déroulant"=w471, "Symphony.lvclass"=w470) -> ("sortie d'erreur"=w468:errorcluster, "Symphony.lvclass Out"=w467:refnum<class "SymphonyCCD.lvclass">)  [unwired: 7 in]
              }
            }
          }
          event "Init Program": Value Change {
            n210 = event-data() -> ("NewVal"=w489:bool)  [unwired: 1 in]
            n211 = case shown="Vrai" w489 {
              tunnel: w488 -> [w491 w515]
              tunnel: [w491 w510] -> w487
              tunnel: w486 -> [w490 w523]
              tunnel: [w490 w512] -> w485
              frame False {
              }
              frame True {
                n212 = property class="SymphonyCCD.lvclass"(reference=w523, error in=w515) -> (reference out=w507:refnum<class "SymphonyCCD.lvclass">, error out=w494:errorcluster, "Accessor:VisaRes"=w511:refnum<visa-resource-name>, "Accessor:DataBindCtrl"=w495:string[])
                n213 = call <userlib>:"Symphony ReadWrite.vi"("Read timeout ms(10000)"=5000, "URL"=w511, "Message In"=cluster{"Message":string, "Data":variant, i32} {"Message"="CheckStatus", "Data"=variant, 0} ("élément"), "ErrorIn (no error)"=w494, "CloseConn"=FALSE) -> ("ServerOut"=w513:refnum<k13>, "ClientOut"=w514:refnum<k13>, "Data Out"=w520:T3, "error out"=w516:errorcluster)  [unwired: 7 in]
                n214 = Unbundle By Name(w507) -> ("LambdaSrc"=w492:string, "LambdaMultiplier"=w493:dbl, "LambdaFactor"=w505:dbl, "LambdaOffset"=w504:dbl, "LambdaSrc"=w506:string)
                n215 = Unbundle By Name(w520) -> ("Message"=w509:string, "Data"=w517:variant)
                n216 = Equal?(x="Status" ("y"), y=w509) -> (x = y?=w519:bool)
                n217 = local write "LambdaOffset"(w504) -> ()
                n218 = local write "MaxFindStart"(w505) -> ()
                n219 = local write "MaxFindEnd"(w493) -> ()
                n220 = case shown="Vrai" w519 {
                  tunnel: w517 -> [_ w558]
                  tunnel: w516 -> [w525 w557]
                  tunnel: [w525 w538] -> w510
                  tunnel: w507 -> [w526 w550]
                  tunnel: w514 -> [_ w549]
                  tunnel: w513 -> [_ w540]
                  tunnel: [w526 w548] -> w512
                  frame False {
                    n221 = One Button Dialog(message="Camera server not responding! Check camera program is running and datasocket server is started " ("y")) -> ()  [unwired: 1 in, 1 out]
                  }
                  frame True {
                    n222 = Variant To Data(error in=w557, type=T5 {"Chaînes et valeurs []"=[], 0, "Chaînes et valeurs [] 2"=[], 0, 0, [], nan, TRUE, TRUE, 0, 0}, Variant=w558) -> (data=w556:T5, error out=w539:errorcluster)
                    n223 = Bundle By Name(cluster=w550, "Server"=w540, "Client"=w549) -> (w548:refnum<class "SymphonyCCD.lvclass">)
                    n224 = Unbundle(w556) -> ("Chaînes et valeurs []"=w554:T4, w555:u16, "Chaînes et valeurs [] 2"=w553:T4, w536:u16, w552:i16, w551:i32[][], w546:dbl, w529:u16, w528:u16)  [unwired: 2 out]
                    n225 = local write "Accumulation"(w529) -> ()
                    n226 = call <userlib>:"Symphony GetProgPar.vi"("Param"=enum16{"InitVal", "Tous"}."Tous", "error in"=w539) -> ("Y Bins"=w543:i32, "X Start"=w542:i32, "X End"=w541:i32, "ImageMode"=w535:bool, "Shutter Enable"=w534:bool, "error out"=w537:errorcluster)  [unwired: 3 in, 5 out]
                    n227 = local write "Noise Mode"(w528) -> ()
                    n228 = property on="ADC" class="MDér (strict)"(error in=w539, "StringsAndValues[]"=w554, "Value"=w555) -> (error out=w547:errorcluster)  [unwired: 1 in, 1 out]
                    n229 = local write "areas"(w551) -> ()
                    n230 = property on="Gain" class="MDér (strict)"(error in=w539, "StringsAndValues[]"=w553, "Value"=w536) -> (error out=w531:errorcluster)  [unwired: 1 in, 1 out]
                    n231 = local write "Temp °C"(w546) -> ()
                    n232 = local write "IntegTime"(w552) -> ()
                    n233 = local write "Y Bins"(w543) -> ()
                    n234 = local write "X Start"(w542) -> ()
                    n235 = local write "X End"(w541) -> ()
                    n236 = local write "Image Mode"(w535) -> ()
                    n237 = local write "Shutter Enable"(w534) -> ()
                    n238 = property on="SetAreas" class="Bool (strict)"(error in=w531, "Val(Sgnl)"=TRUE ("Valeur (Signalisation)")) -> (error out=w533:errorcluster)  [unwired: 1 in, 1 out]
                    n239 = property on="Shutter Enable" class="Bool (strict)"(error in=w533, "Val(Sgnl)"=w534) -> (error out=w532:errorcluster)  [unwired: 1 in, 1 out]
                    n240 = Merge Errors(w537, w547, w531, w532) -> (w538:errorcluster)
                  }
                }
                n241 = Search 1D Array(1D array=w495, element=w506) -> (index of element=w502:i32)  [unwired: 1 in]
                n242 = Search 1D Array(1D array=w495, element=w492) -> (index of element=w497:i32)  [unwired: 1 in]
                n243 = Greater Or Equal To 0?(x=w502) -> (x >= 0?=w503:bool)
                n244 = Greater Or Equal To 0?(x=w497) -> (x >= 0?=w496:bool)
                n245 = Select(t=w502, s=w503, f=0 ("cas faux")) -> (s? t:f=w501:i32)
                n246 = Select(t=w497, s=w496, f=0 ("cas faux")) -> (s? t:f=w498:i32)
                n247 = property on="Wavelength Source" class="MDér (strict)"(error in=w494, "Strings []"=w495, "Value"=w501) -> ()  [unwired: 1 in, 2 out]
                n248 = property on="MultSource" class="MDér (strict)"(error in=w494, "Strings []"=w495, "Value"=w498) -> ()  [unwired: 1 in, 2 out]
                "Init Program" <- FALSE
              }
            }
          }
          event "Tabs": Value Change {
            n249 = event-data() -> ("NewVal"=w563:T1)  [unwired: 1 in, 5 out]
            n250 = case shown="\"Areas\"" w563 {
              tunnel: w562 -> [w565 w567 w579]
              tunnel: w561 -> [w564 w566 w581]
              tunnel: [w565 w567 w580] -> w560
              tunnel: [w564 w566 w570] -> w559
              frame "Main Settings", Default {
              }
              frame "Areas" {
              }
              frame "Conversion & Settings" {
                n251 = Unbundle By Name(w579) -> ("LambdaSrc"=w578:string, "MultiplierSrc"=w572:string)
                n252 = property class="SymphonyCCD.lvclass"(reference=w579, error in=w581) -> (reference out=w580:refnum<class "SymphonyCCD.lvclass">, error out=w568:errorcluster, "Accessor:DataBindCtrl"=w571:string[])
                n253 = Search 1D Array(1D array=w571, element=w572) -> (index of element=w575:i32)  [unwired: 1 in]
                n254 = Search 1D Array(1D array=w571, element=w578) -> (index of element=w584:i32)  [unwired: 1 in]
                n255 = Greater Or Equal To 0?(x=w575) -> (x >= 0?=w574:bool)
                n256 = Greater Or Equal To 0?(x=w584) -> (x >= 0?=w585:bool)
                n257 = Select(t=w575, s=w574, f=0 ("cas faux")) -> (s? t:f=w573:i32)
                n258 = Select(t=w584, s=w585, f=0 ("cas faux")) -> (s? t:f=w583:i32)
                n259 = property on="MultSource" class="MDér (strict)"(error in=w568, "Strings []"=w571, "Value"=w573) -> (error out=w569:errorcluster)  [unwired: 1 in, 1 out]
                n260 = property on="Wavelength Source" class="MDér (strict)"(error in=w568, "Strings []"=w571, "Value"=w583) -> (error out=w577:errorcluster)  [unwired: 1 in, 1 out]
                n261 = Merge Errors(w569, w577) -> (w570:errorcluster)
              }
            }
          }
        }
        n262 = Or(x=w84, y="Stop") -> (x .or. y?=w82:bool)
      }
    }
    frame Error {
    }
  }
  "error out" <- w5
  "SymphonyCCD.lvclass Out" <- w3
